vi "Set Output.vi"(8 "error in (no error)":errorcluster {"code" format="%.0x"}, 9 "TriggerType (HSWP)":i32(ring) items=["HSWP", "Measuring", "Main", "Gate", "G Trigger", "O Even", "SU Video", "SSettled", "S1 Marker", "S2 Marker", "S3 Marker", "S4 Marker", "OFF", "S Point"], 10 "RearTriggerNo":i32=1 format="%.0g", 11 "instrument handle":refnum<k15>) -> (0 "error out":errorcluster {"code" format="%.0x"}, 3 "instrument handle out":refnum<k15>)   [LabVIEW 2021, in "Keysight XSAnVMA.lvlib"]
doc: "Returns the type of output signal that will be output from the rear panel Trigger 1 Out connector."
uses:
  <instrlib>/Keysight XSAnVMA/Keysight XSAnVMA.lvlib
  KtXSAnVMA_64.dll
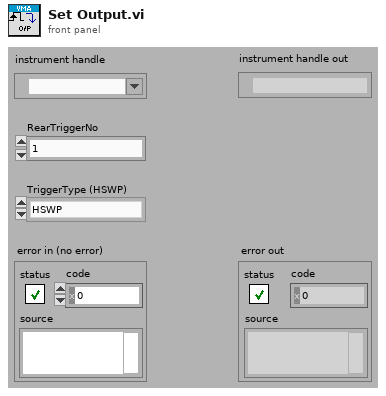
[diagram p1: front panel]
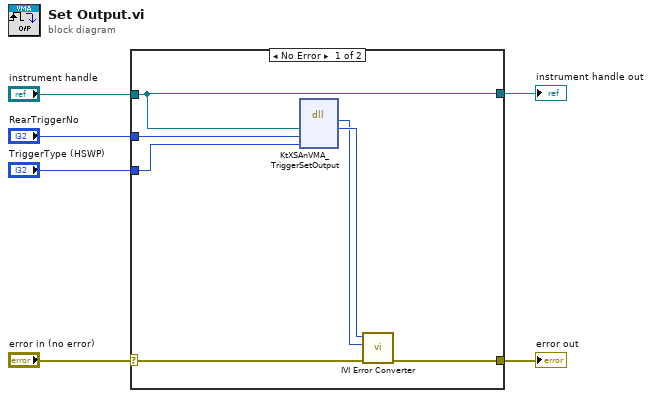
[diagram p0: block diagram]
diagram:
  n1 = case shown="No Error" "error in (no error)" {
    selector: "error in (no error)" -> [w11 w15]
    tunnel: [w10 w15] -> w6
    tunnel: "instrument handle" -> [w7 w14]
    tunnel: "RearTriggerNo" -> [w9 _]
    tunnel: "TriggerType (HSWP)" -> [w8 _]
    tunnel: [w7 w14] -> w1
    frame No Error {
      n2 = dll-call lib="KtXSAnVMA**.dll" fn="KtXSAnVMA_TriggerSetOutput"("Vi"=w7, "RearTriggerNo"=w9, "TriggerType"=w8) -> (w12:i32, "Vi"=w13:u32)  [unwired: 5 in, 2 out]
      n3 = call <instrlib>:"IVI Error Converter.vi"("error in (no error)"=w11, "IVI error code (0)"=w12, "instrument handle"=w13) -> ("error out"=w10:errorcluster)  [unwired: 7 in, 1 out]
    }
    frame Error {
    }
  }
  "error out" <- w6
  "instrument handle out" <- w1
